vi "Msg To.vi"() -> (3 "Teardown Msg Strategy out":refnum<class "Teardown Msg Strategy.lvclass">)   [LabVIEW 2021, in "jettl.lvlib" / "Teardown.lvlib"]
uses:
  Teardown.lvlib
  Teardown Msg Strategy/Teardown Msg Strategy.lvclass
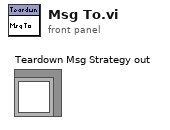
[diagram p1: front panel]
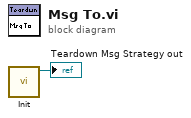
[diagram p0: block diagram]
diagram:
  n1 = call "Init.vi"() -> ("Teardown Msg Strategy out"=→"Teardown Msg Strategy out":refnum<class "Teardown Msg Strategy.lvclass">)  [unwired: 11 in]
